vi "FGV_TEST(subvi).vi"(2 "error in (no error)":errorcluster caption="에러 입력(에러 없음)", 3 "상태컨트롤":enum16{"초기화", "읽기", "쓰기"}(ring), 4 "IN":dbl) -> (0 "error out":errorcluster caption="에러 출력", 1 "OUT":dbl)   [LabVIEW 2020]
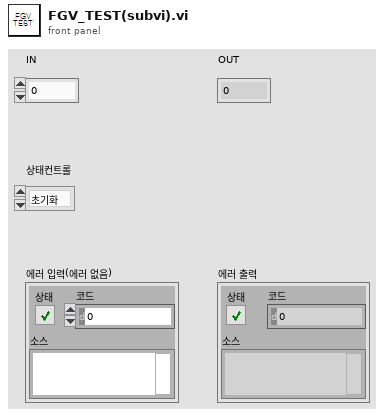
[diagram p1: front panel]
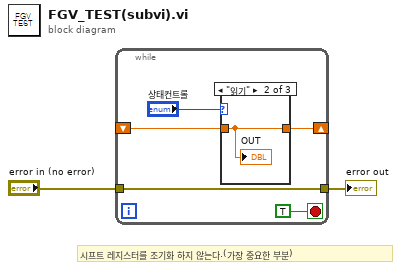
[diagram p0: block diagram]
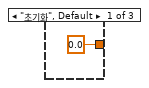
[diagram p2: hidden frame]
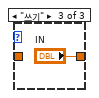
[diagram p3: hidden frame]
diagram:
  # "시프트 레지스터를 조기화 하지 않는다.(가장 중요한 부분)"
  n1 = while {
    shift-right: [w4] -> _
    shift-left: _ -> [w5]
    tunnel: [w6] -> w1
    tunnel: "error in (no error)" -> [w6]
    stop <- TRUE stop-if-true
    n2 = case shown="\"읽기\"" "상태컨트롤" {
      tunnel: w5 -> [_ w9 _]
      tunnel: [0.0 ("숫자형") w9 "IN"] -> w4
      frame "초기화", Default {
      }
      frame "읽기" {
        "OUT" <- w9
      }
      frame "쓰기" {
      }
    }
  }
  "error out" <- w1
